vi "File Path Suffix.vi"(8 "Data file type":string, 9 "Suffix string":string, 10 "File type":string, 11 "File path":path) -> (3 "New file path":path)   [LabVIEW 2020]
panel:
  in  "Tab Control":enum32{"Input", "Output"}(tab)
  # "Description:\nAdds suffix to file name with same file type and file path."
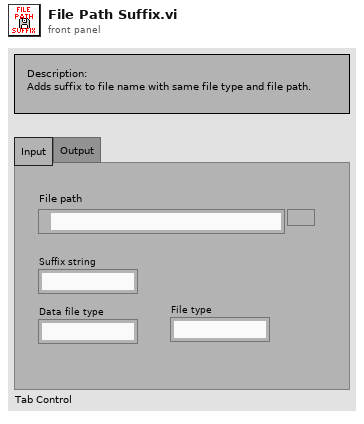
[diagram p1: front panel]
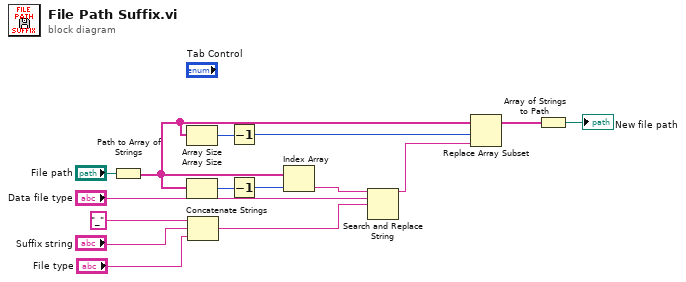
[diagram p0: block diagram]
diagram:
  n1 = Path to Array of Strings(0:"File path") -> (2:w10:string[])  [unwired: 1 out]
  n2 = Array Size(array=w10) -> (size(s)=w12:i32)
  n3 = Array Size(array=w10) -> (size(s)=w14:i32)
  n4 = Concatenate Strings("_" ("string"), "Suffix string", "File type") -> (w4:string)
  n5 = Decrement(x=w12) -> (x-1=w11:i32)
  n6 = Decrement(x=w14) -> (x-1=w13:i32)
  n7 = Index Array(array=w10, index=w13) -> (element=w5:string)
  n8 = Search and Replace String(input string=w5, search string="Data file type", replace string=w4) -> (result string=w2:string)  [unwired: 5 in, 3 out]
  n9 = Replace Array Subset(array=w10, new element=w2, index=w11) -> (w9:string[])
  n10 = Array of Strings to Path(0:w9) -> (2:→"New file path":path)  [unwired: 1 in]
